vi "Comments.vi"() -> ()   [LabVIEW 2020]
panel:
  out "x+y":dbl
  in  "x":dbl
  in  "y":dbl
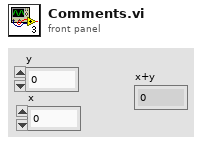
[diagram p1: front panel]
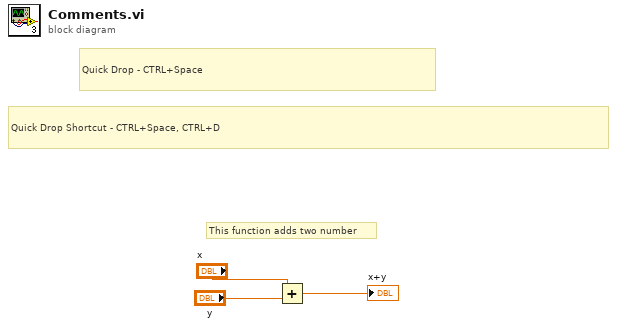
[diagram p0: block diagram]
diagram:
  # "Quick Drop Shortcut - CTRL+Space, CTRL+D"
  # "Quick Drop - CTRL+Space"
  # "This function adds two number"
  n1 = Add(x="x", y="y") -> (x+y=→"x+y":dbl)
